vi "调整内边框位置.vi"(8 "错误输入（无错误）":errorcluster, 10 "位置":cluster{"left":i16, "top":i16}, 11 "引用":refnum<vi>) -> (0 "错误输出":errorcluster, 3 "引用输出":refnum<vi>)   [LabVIEW 8.6, in "窗口操作.lvlib"]
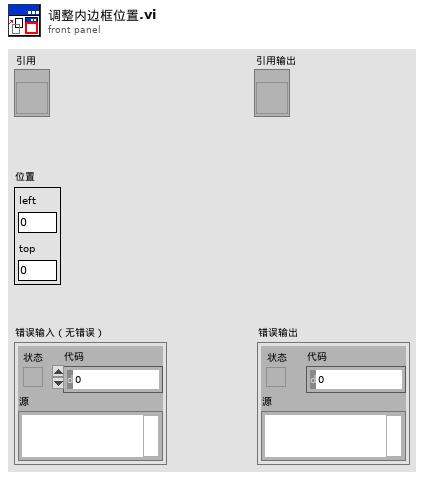
[diagram p1: front panel]
types:
  T1 = typedef "LVRectTypeDef.ctl" = cluster{"Left":i16, "Top":i16, "Right":i16, "Bottom":i16}
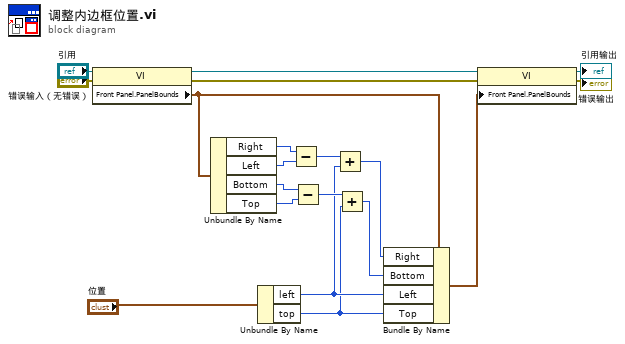
[diagram p0: block diagram]
diagram:
  n1 = property class="VI"(reference="引用", error in="错误输入（无错误）") -> (reference out=w6:refnum<vi>, error out=w7:errorcluster, "Front Panel.PanelBounds"=w18:T1)
  n2 = Unbundle By Name(w18) -> ("Right"=w16:i16, "Left"=w17:i16, "Bottom"=w15:i16, "Top"=w14:i16)
  n3 = Unbundle By Name("位置") -> ("left"=w9:i16, "top"=w8:i16)
  n4 = Subtract(x=w16, y=w17) -> (x-y=w13:i16)
  n5 = Subtract(x=w15, y=w14) -> (x-y=w12:i16)
  n6 = Add(x=w13, y=w9) -> (x+y=w10:i16)
  n7 = Add(x=w12, y=w8) -> (x+y=w11:i16)
  n8 = Bundle By Name(cluster=w18, "Right"=w10, "Bottom"=w11, "Left"=w9, "Top"=w8) -> (w19:T1)
  n9 = property class="VI"(reference=w6, error in=w7, "Front Panel.PanelBounds"=w19) -> (reference out=→"引用输出":refnum<vi>, error out=→"错误输出":errorcluster)
